vi "Event Handle Loop.vi"(8 "error in (no error)":errorcluster, 11 "QMenu Class in":refnum<class "QMenu Class.lvclass">) -> (0 "error out":errorcluster, 3 "QMenu Class out":refnum<class "QMenu Class.lvclass">)   [LabVIEW 2020, in "QTab.lvlib" / "QMenu Class.lvclass"]
uses:
  QMenu Class.lvclass
  Command.ctl
  QMenu Class.lvclass/QMenu Class.ctl
  Button Attribute.ctl
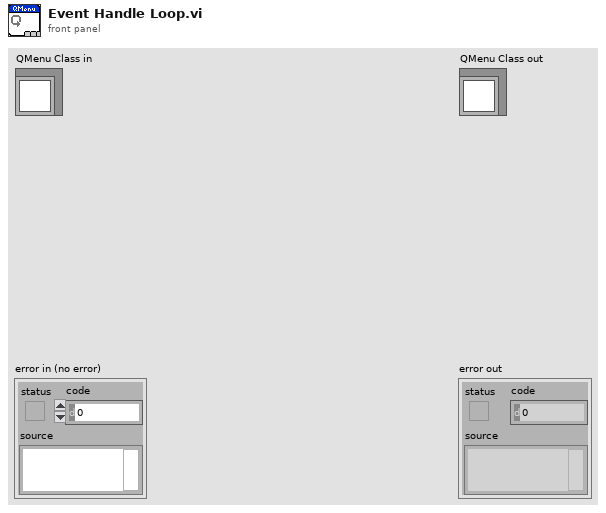
[diagram p1: front panel]
types:
  T1 = typedef "QTab.lvlib/QMenu Class.lvclass/Command.ctl" = enum16{"Initialize", "Get Active Button", "Set Active Button", "Set Button Attribute", "Add Button", "Close Button", "Draw", "Stop"}
  T2 = typedef "QTab.lvlib/QMenu Class.lvclass/Button Attribute.ctl" = cluster{"Label":string, "Button Text":string, "Closable":bool, "Draggable":bool}
  T3 = typedef "LVPoint32TypeDef.ctl" = cluster{"Horizontal":i32, "Vertical":i32}
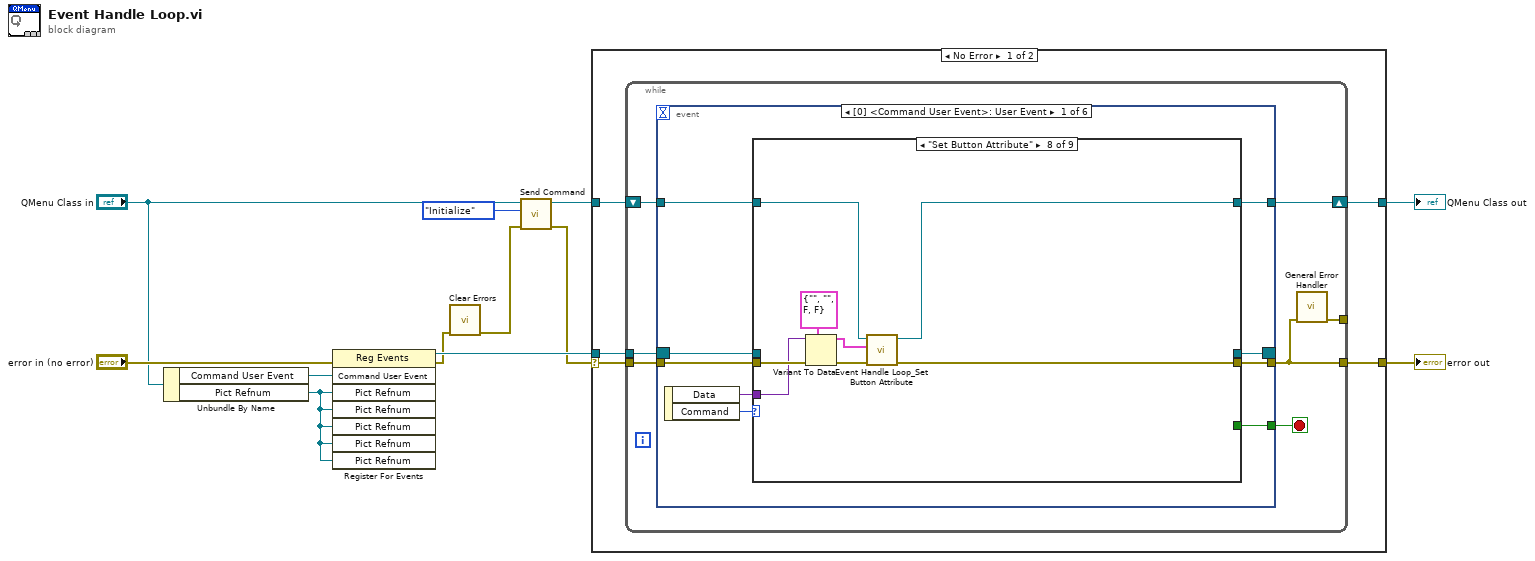
[diagram p0: block diagram]
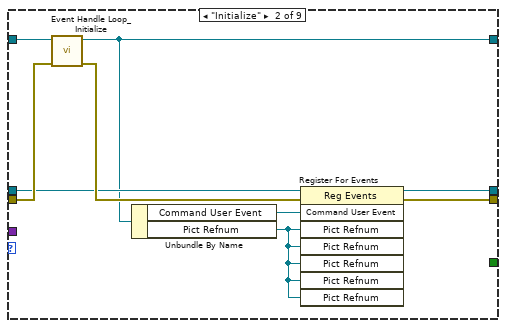
[diagram p3: hidden frame]
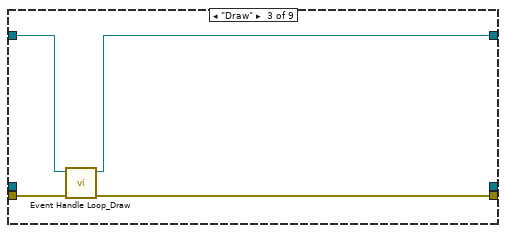
[diagram p4: hidden frame]
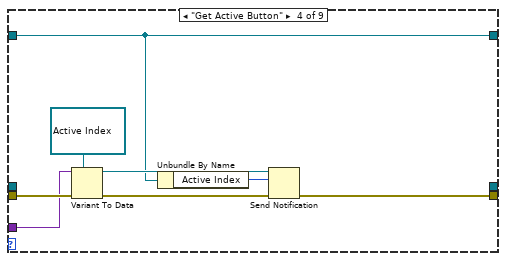
[diagram p5: hidden frame]
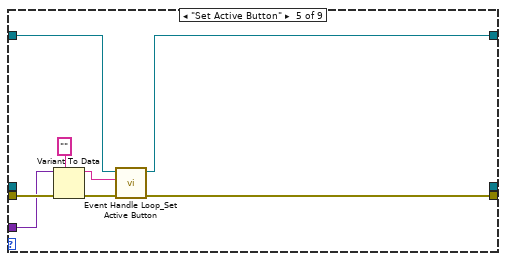
[diagram p6: hidden frame]
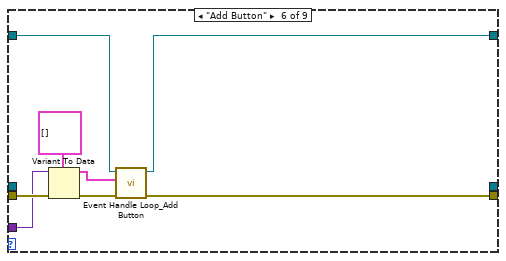
[diagram p7: hidden frame]
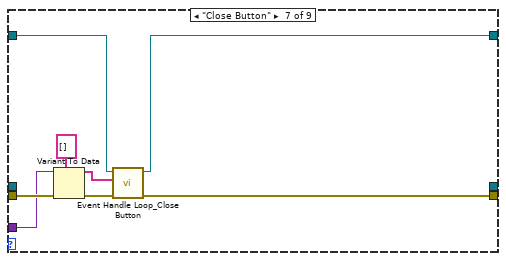
[diagram p8: hidden frame]
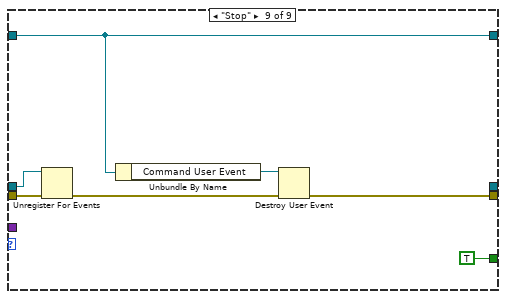
[diagram p9: hidden frame]
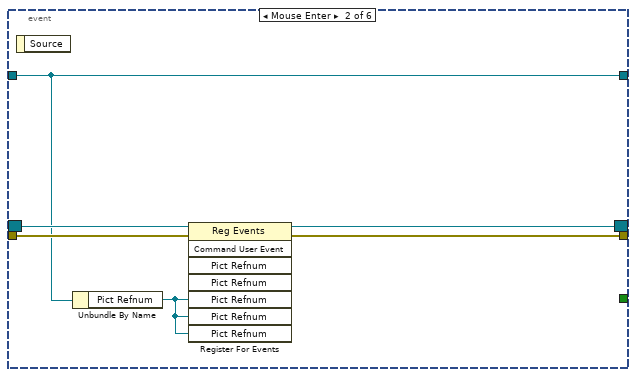
[diagram p10: hidden frame]
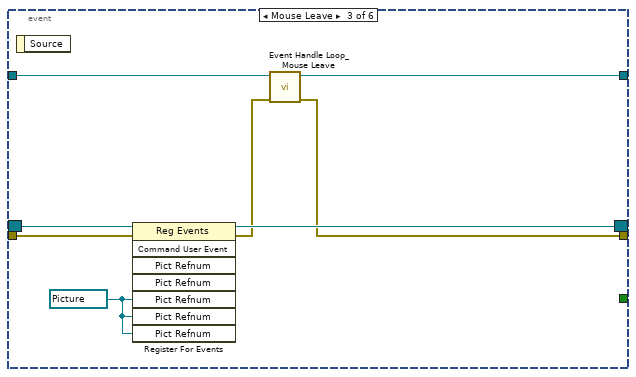
[diagram p11: hidden frame]
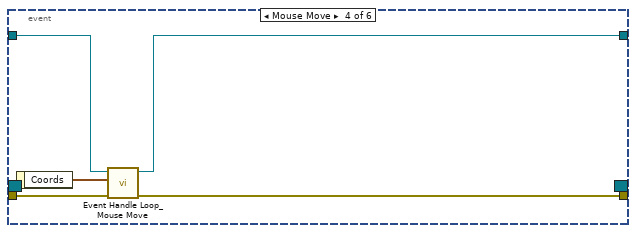
[diagram p12: hidden frame]
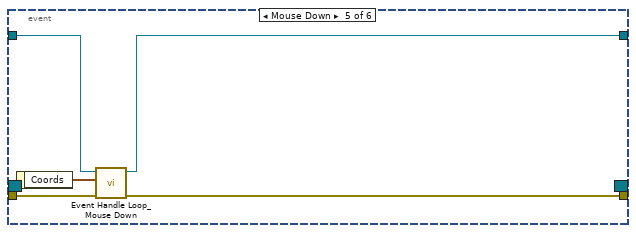
[diagram p13: hidden frame]
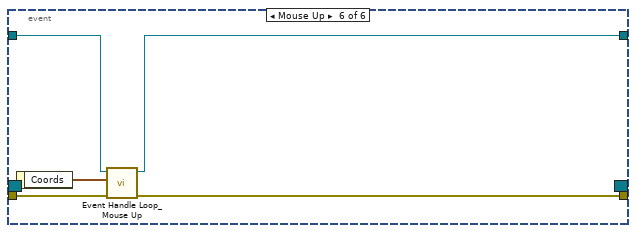
[diagram p14: hidden frame]
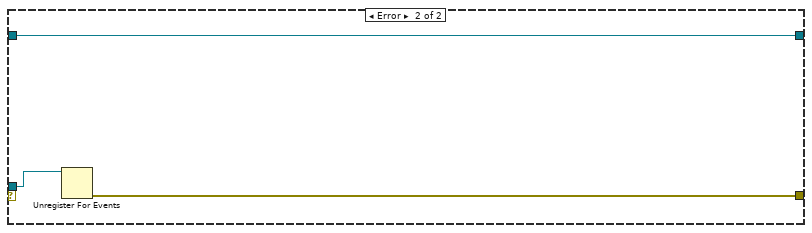
[diagram p15: hidden frame]
diagram:
  n1 = Unbundle By Name("QMenu Class in") -> ("Command User Event"=w10:refnum<user-event>, "Pict Refnum"=w3:refnum<vi>)
  n2 = register-events(error in="error in (no error)", w10, w3, w3, w3, w3, w3) -> (reference out=w11:refnum<event-registration>, error out=w2:errorcluster)  [unwired: 1 in]
  n3 = call <vilib>:"Clear Errors.vi"("error in (no error)"=w2) -> ("error out"=w1:errorcluster)  [unwired: 5 in, 1 out]
  n4 = call "Send Command.vi"("error in (no error)"=w1, "Command"=Command."Initialize", "QMenu Class in"="QMenu Class in") -> ("error out"=w4:errorcluster, "QMenu Class out"=w8:refnum<class "QMenu Class.lvclass">)  [unwired: 7 in]
  n5 = case shown="No Error" w4 {
    selector: w4 -> [w13 _]
    tunnel: w11 -> [w17 w128]
    tunnel: w8 -> [w16 w126]
    tunnel: [w15 w126] -> w6
    tunnel: [w14 w127] -> w5
    frame No Error {
      n6 = while {
        tunnel: w13 -> [w24]
        tunnel: w17 -> [w23]
        tunnel: [w19] -> w14
        shift-right: [w21] -> w15
        shift-left: w16 -> [w22]
        tunnel: [w18] -> _
        stop <- w20 stop-if-true
        n7 = event shown="[0] <Command User Event>: User Event" {
          selector: w23 -> [w30 w101 w109 _ _ _]
          dyn-events: [w25 w99 w108 _ _ _] -> _
          timeout: _ -> [_ _ _ _ _ _]
          tunnel: w24 -> [w31 w102 w110 w115 w120 w125]
          tunnel: w22 -> [w29 w98 w103 w113 w118 w124]
          tunnel: [w28 w98 w105 w112 w117 w123] -> w21
          tunnel: [w27 w100 w104 w111 w116 w122] -> w19
          tunnel: [w26 _ _ _ _ _] -> w20
          event User Event {
            n8 = event-data() -> ("Data"=w32:variant, "Command"=w33:T1)  [unwired: 1 in]
            n9 = case shown="\"Set Button Attribute\"" w33 {
              tunnel: w32 -> [_ _ _ w55 w64 w72 w80 w88 _]
              tunnel: w31 -> [w35 w45 w49 w57 w65 w73 w81 w89 w96]
              tunnel: w30 -> [w34 w39 _ _ _ _ _ _ w95]
              tunnel: w29 -> [w36 w44 w48 w51 w60 w68 w77 w84 w93]
              tunnel: [w36 w37 w47 w51 w59 w67 w76 w83 w93] -> w28
              tunnel: [w35 w40 w46 w52 w58 w66 w75 w82 w90] -> w27
              tunnel: [_ _ _ _ _ _ _ _ TRUE] -> w26
              tunnel: [w34 w38 _ _ _ _ _ _ _] -> w25
              frame Default {
              }
              frame "Initialize" {
                n10 = call "Event Handle Loop_Initialize.vi"("error in (no error)"=w45, "QMenu Class in"=w44) -> ("error out"=w41:errorcluster, "QMenu Class out"=w37:refnum<class "QMenu Class.lvclass">)  [unwired: 8 in]
                n11 = Unbundle By Name(w37) -> ("Command User Event"=w43:refnum<user-event>, "Pict Refnum"=w42:refnum<vi>)
                n12 = register-events(reference=w39, error in=w41, w43, w42, w42, w42, w42, w42) -> (reference out=w38:refnum<event-registration>, error out=w40:errorcluster)
              }
              frame "Draw" {
                n13 = call "Event Handle Loop_Draw.vi"("error in (no error)"=w49, "QMenu Class in"=w48) -> ("error out"=w46:errorcluster, "QMenu Class out"=w47:refnum<class "QMenu Class.lvclass">)  [unwired: 8 in]
              }
              frame "Get Active Button" {
                n14 = Variant To Data(error in=w57, type=refnum<notifier> refnum ("notifier out"), Variant=w55) -> (data=w53:refnum<notifier>, error out=w54:errorcluster)
                n15 = Unbundle By Name(w51) -> ("Active Index"=w50:i32)
                n16 = Send Notification(notification=w50, notifier=w53, error in (no error)=w54) -> (error out=w52:errorcluster)  [unwired: 1 out]
              }
              frame "Set Active Button" {
                n17 = Variant To Data(error in=w65, type="", Variant=w64) -> (data=w61:string, error out=w62:errorcluster)
                n18 = call "Event Handle Loop_Set Active Button.vi"("error in (no error)"=w62, "Label"=w61, "QMenu Class in"=w60) -> ("error out"=w58:errorcluster, "QMenu Class out"=w59:refnum<class "QMenu Class.lvclass">)  [unwired: 7 in]
              }
              frame "Add Button" {
                n19 = Variant To Data(error in=w73, type=T2[] [] ("Button Attribute []"), Variant=w72) -> (data=w69:T2[], error out=w70:errorcluster)
                n20 = call "Event Handle Loop_Add Button.vi"("error in (no error)"=w70, "Button Attribute []"=w69, "QMenu Class in"=w68) -> ("error out"=w66:errorcluster, "QMenu Class out"=w67:refnum<class "QMenu Class.lvclass">)  [unwired: 7 in]
              }
              frame "Close Button" {
                n21 = Variant To Data(error in=w81, type=string[] [], Variant=w80) -> (data=w74:string[], error out=w78:errorcluster)
                n22 = call "Event Handle Loop_Close Button.vi"("error in (no error)"=w78, "Label"=w74, "QMenu Class in"=w77) -> ("error out"=w75:errorcluster, "QMenu Class out"=w76:refnum<class "QMenu Class.lvclass">)  [unwired: 7 in]
              }
              frame "Set Button Attribute" {
                n23 = Variant To Data(error in=w89, type=T2 {"Label"="", "Button Text"="", "Closable"=FALSE, "Draggable"=FALSE} ("Button Attribute"), Variant=w88) -> (data=w85:T2, error out=w86:errorcluster)
                n24 = call "Event Handle Loop_Set Button Attribute.vi"("error in (no error)"=w86, "Button Attribute"=w85, "QMenu Class in"=w84) -> ("error out"=w82:errorcluster, "QMenu Class out"=w83:refnum<class "QMenu Class.lvclass">)  [unwired: 7 in]
              }
              frame "Stop" {
                n25 = Unregister For Events(event registration refnum=w95, error in=w96) -> (error out=w92:errorcluster)
                n26 = Unbundle By Name(w93) -> ("Command User Event"=w91:refnum<user-event>)
                n27 = Destroy User Event(user event=w91, error in=w92) -> (error out=w90:errorcluster)
              }
            }
          }
          event Mouse Enter {
            n28 = event-data() -> ()  [unwired: 1 in, 1 out]
            n29 = Unbundle By Name(w98) -> ("Pict Refnum"=w97:refnum<vi>)
            n30 = register-events(reference=w101, error in=w102, w97, w97, w97) -> (reference out=w99:refnum<event-registration>, error out=w100:errorcluster)  [unwired: 3 in]
          }
          event Mouse Leave {
            w107 = refnum<vi> refnum ("event source")
            n31 = event-data() -> ()  [unwired: 1 in, 1 out]
            n32 = register-events(reference=w109, error in=w110, w107, w107, w107) -> (reference out=w108:refnum<event-registration>, error out=w106:errorcluster)  [unwired: 3 in]
            n33 = call "Event Handle Loop_Mouse Leave.vi"("error in (no error)"=w106, "QMenu Class in"=w103) -> ("error out"=w104:errorcluster, "QMenu Class out"=w105:refnum<class "QMenu Class.lvclass">)  [unwired: 8 in]
          }
          event Mouse Move {
            n34 = event-data() -> ("Coords"=w114:T3)  [unwired: 1 in]
            n35 = call "Event Handle Loop_Mouse Move.vi"("error in (no error)"=w115, "Coords"=w114, "QMenu Class in"=w113) -> ("error out"=w111:errorcluster, "QMenu Class out"=w112:refnum<class "QMenu Class.lvclass">)  [unwired: 7 in]
          }
          event Mouse Down {
            n36 = event-data() -> ("Coords"=w119:T3)  [unwired: 1 in]
            n37 = call "Event Handle Loop_Mouse Down.vi"("error in (no error)"=w120, "Coords"=w119, "QMenu Class in"=w118) -> ("error out"=w116:errorcluster, "QMenu Class out"=w117:refnum<class "QMenu Class.lvclass">)  [unwired: 7 in]
          }
          event Mouse Up {
            n38 = event-data() -> ("Coords"=w121:T3)  [unwired: 1 in]
            n39 = call "Event Handle Loop_Mouse Up.vi"("error in (no error)"=w125, "Coords"=w121, "QMenu Class in"=w124) -> ("error out"=w122:errorcluster, "QMenu Class out"=w123:refnum<class "QMenu Class.lvclass">)  [unwired: 7 in]
          }
        }
        n40 = call <vilib>:"General Error Handler.vi"("error in (no error)"=w19) -> ("error out"=w18:errorcluster)  [unwired: 10 in, 4 out]
      }
    }
    frame Error {
      n41 = Unregister For Events(event registration refnum=w128) -> (error out=w127:errorcluster)  [unwired: 1 in]
    }
  }
  "error out" <- w5
  "QMenu Class out" <- w6
